vi "GE 5565PIORC.String Buffer.vi"(8 "error in (no error)":errorcluster, 9 "string buffer in":string, 10 "minimum size":i32, 11 "GE 5565PIORC in":refnum<class "GE 5565PIORC.lvclass">) -> (0 "error out":errorcluster, 1 "string buffer out":string, 3 "GE 5565PIORC out":refnum<class "GE 5565PIORC.lvclass">)   [LabVIEW 2024, in "GE 5565PIORC.lvclass"]
uses:
  GE 5565PIORC.lvclass
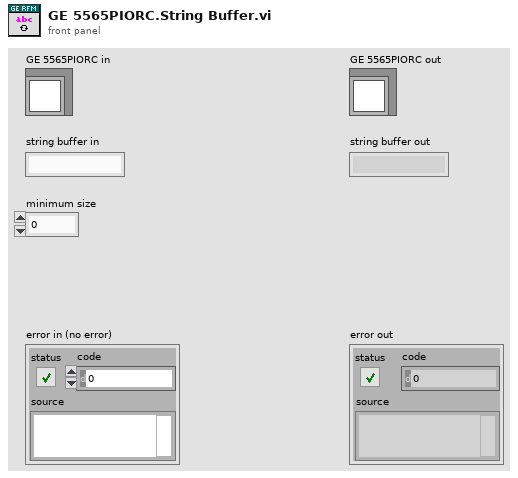
[diagram p1: front panel]
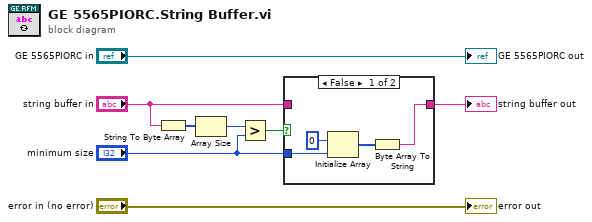
[diagram p0: block diagram]
diagram:
  n1 = String To Byte Array(string="string buffer in") -> (unsigned byte array=w6:u8[])
  n2 = Array Size(array=w6) -> (size(s)=w1:i32)
  n3 = Greater?(x=w1, y="minimum size") -> (0:w5:bool)
  n4 = case shown="False" w5 {
    tunnel: "string buffer in" -> [_ w13]
    tunnel: "minimum size" -> [w11 _]
    tunnel: [w9 w13] -> w2
    frame False {
      n5 = Initialize Array(u8 0 ("element"), w11) -> (w10:u8[])
      n6 = Byte Array To String(unsigned byte array=w10) -> (string=w9:string)
    }
    frame True {
    }
  }
  "string buffer out" <- w2
  "GE 5565PIORC out" <- "GE 5565PIORC in"
  "error out" <- "error in (no error)"
